vi "GetOverlay.vi"(8 "error in":errorcluster, 11 "Abstract Engine":refnum<class "Abstract Engine.lvclass">) -> (0 "error out":errorcluster, 2 "overlay":string, 3 "Abstract Engine out":refnum<class "Abstract Engine.lvclass">)   [LabVIEW 2025, in "Abstract Engine.lvlib" / "Abstract Engine.lvclass"]
doc: "Copyright 2017 National Instruments Corporation\n\nLicensed under the Apache License, Version 2.0 (the \"License\"); you may not use this file except in compliance with the License. You may obtain a copy of the License at http://www.apache.org/licenses/LICENSE-2.0\nUnless required by applicable law or agreed to in writing, software distributed under the License is distributed on an \"AS IS\" BASIS, WITHOUT WARRANTIES OR CONDITIONS OF ANY KIND, either express or implied. See the License for the specific language governing permissions and limitations under the License."
uses:
  Abstract Engine.lvclass
  Abstract Engine.lvclass/Abstract Engine.ctl
  Users/Public/Documents/Sandia National Labs/TSS Plugin/CEF.lvlibp/serializable node/CEF_serializable node.lvclass
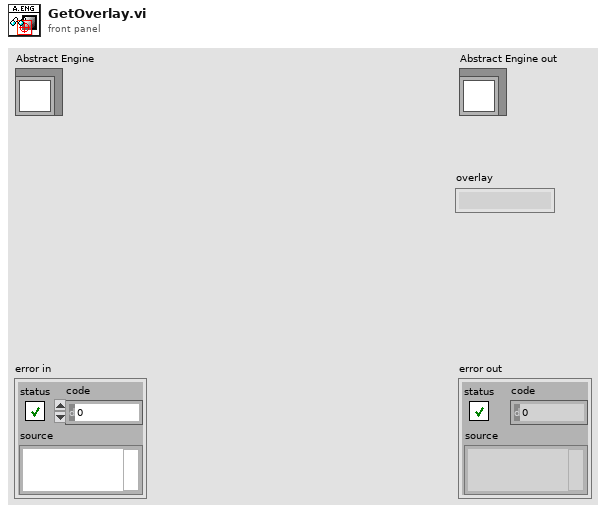
[diagram p1: front panel]
types:
  T1 = typedef "Abstract Engine.lvlib/Abstract Engine.lvclass/Engine Cluster.ctl" = cluster{"IP Address":string, "Type":string, "Initialized":bool, "InstrumentMap":map{string, cluster{"Initialized":bool, "Channels":T2[]}}}
  T2 = typedef "Abstract Engine.lvlib/Abstract Instrument.lvclass/Channel.ctl" = cluster{"Alias":string, "Type":enum16{"Numeric", "Boolean", "String"}, "Unit":T3, "Upper limit":dbl, "Lower limit":dbl, "Measurement":variant}
  T3 = typedef "Abstract Engine.lvlib/Abstract Instrument.lvclass/Unit.ctl" = enum16{"---", "V", "A", "Ohm", "Hz", "uF", "degC", "deg"}
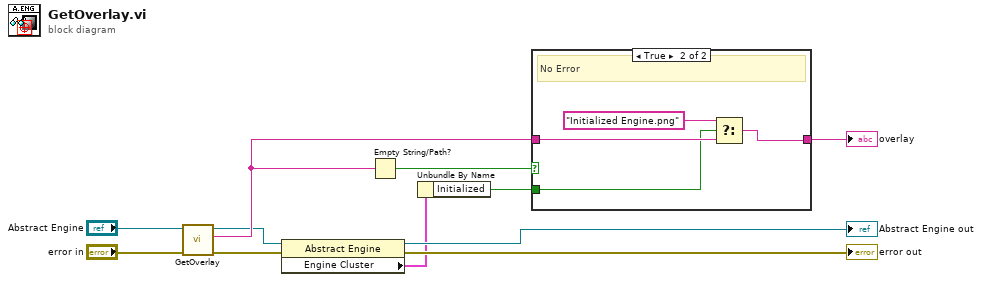
[diagram p0: block diagram]
diagram:
  n1 = call-parent "GetOverlay.vi"("error in"="error in", "CEF_serializable node in"="Abstract Engine") -> ("error out"=w5:errorcluster, "overlay"=w8:string, "CEF_serializable node out"=w6:refnum<class "Abstract Engine.lvclass">)  [unwired: 7 in]
  n2 = property class="Abstract Engine"(reference=w6, error in=w5) -> (reference out=→"Abstract Engine out":refnum<class "Abstract Engine.lvclass">, error out=→"error out":errorcluster, "Engine Cluster"=w2:T1)
  n3 = Empty String/Path?(string/path=w8) -> (empty?=w9:bool)
  n4 = Unbundle By Name(w2) -> ("Initialized"=w1:bool)
  n5 = case shown="True" w9 {
    tunnel: w8 -> [w12 w15]
    tunnel: [w12 w14] -> w7
    tunnel: w1 -> [_ w13]
    frame False {
      # "Error pic"
    }
    frame True {
      # "No Error"
      n6 = Select(t="Initialized Engine.png" ("overlay"), s=w13, f=w15) -> (s? t:f=w14:string)
    }
  }
  "overlay" <- w7
